vi "Wait for Message.vi"(8 "error in":errorcluster, 10 "Timeout":i32 format="%d ms", 11 "Read Event in":refnum<class "Read Event.lvclass">) -> (0 "error out":errorcluster, 2 "Timed Out":bool, 3 "Read Event out":refnum<class "Read Event.lvclass">)   [LabVIEW 2019, in "PCANBasic.lvlib" / "Read Event.lvclass"]
uses:
  Read Event.lvclass
  Read Event.lvclass/Read Event.ctl
  Message Waiter/Message Waiter.lvclass
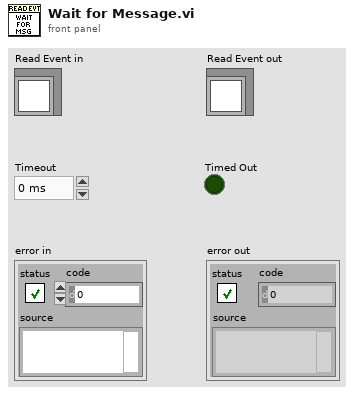
[diagram p1: front panel]
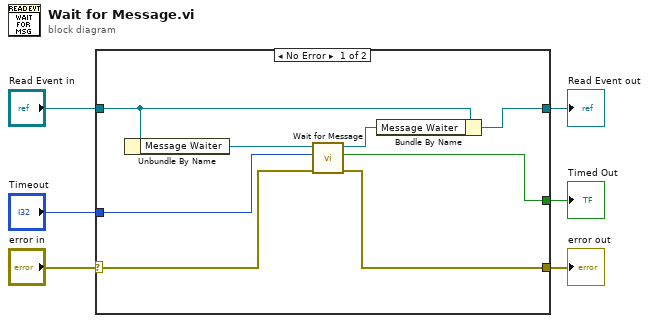
[diagram p0: block diagram]
diagram:
  n1 = case shown="No Error" "error in" {
    selector: "error in" -> [w14 w16]
    tunnel: [w13 w16] -> w5
    tunnel: [w7 w15] -> w3
    tunnel: "Read Event in" -> [w9 w15]
    tunnel: "Timeout" -> [w12 _]
    tunnel: [w11 _] -> w1
    frame No Error {
      n2 = Unbundle By Name(w9) -> ("Message Waiter"=w10:refnum<class "Message Waiter.lvclass">)
      n3 = call-dynamic "Wait for Message.vi"("error in"=w14, "Timeout"=w12, "Message Waiter in"=w10) -> ("error out"=w13:errorcluster, "Timed Out"=w11:bool, "Message Waiter out"=w8:refnum<class "Message Waiter.lvclass">)  [unwired: 6 in]
      n4 = Bundle By Name(cluster=w9, "Message Waiter"=w8) -> (w7:refnum<class "Read Event.lvclass">)
    }
    frame Error {
    }
  }
  "error out" <- w5
  "Read Event out" <- w3
  "Timed Out" <- w1
